vi "Check VI has Action Input.vi"(11 "Worker VI":refnum<vi>) -> (3 "Action Input?":bool)   [LabVIEW 2020, in "FlexBlock.xnode"]
uses:
  FlexBlock.xnode
  FlexBlocks/Worker Action.ctl
  FlexBlocks/FlexBlocks.lvlib
  <vilib>/Utility/Data Type/NI_Data Type.lvlib
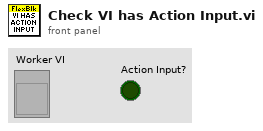
[diagram p1: front panel]
types:
  T1 = typedef "FlexBlocks.lvlib/Worker Action.ctl" = enum16{"Start", "Work", "Stop"}
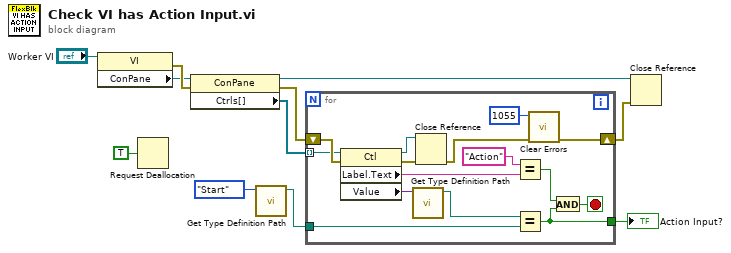
[diagram p0: block diagram]
diagram:
  n1 = property class="VI"(reference="Worker VI") -> (error out=w11:errorcluster, "ConPane"=w9:refnum<vi>)  [unwired: 1 in, 1 out]
  n2 = Request Deallocation(TRUE ("flag")) -> ()
  n3 = property class="ConPane"(reference=w9, error in=w11) -> (reference out=w4:refnum<vi>, error out=w7:errorcluster, "Ctrls[]"=w8:refnum<vi>[])
  n4 = call <vilib>:"Get Type Definition Path.vi"("variant"=Worker_Action."Start" ("Action")) -> ("type definition path"=w2:path)  [unwired: 9 in, 1 out]
  n5 = for {
    tunnel: w2 -> [w24]
    tunnel: w8 -> [w25] mode=indexing
    shift-right: [w13] -> w5
    shift-left: w7 -> [w26]
    tunnel: [w19] -> w6
    stop <- w17 stop-if-true
    n6 = property class="Ctl"(reference=w25, error in=w26) -> (reference out=w22:refnum<vi>, error out=w23:errorcluster, "Label.Text"=w21:string, "Value"=w16:variant)
    n7 = call <vilib>:"Get Type Definition Path.vi"("variant"=w16) -> ("type definition path"=w15:path)  [unwired: 9 in, 1 out]
    n8 = Close Reference(reference=w22, error in (no error)=w23) -> (error out=w14:errorcluster)
    n9 = Equal?(x="Action", y=w21) -> (x = y?=w18:bool)
    n10 = Equal?(x=w15, y=w24) -> (x = y?=w19:bool)
    n11 = call <vilib>:"Clear Errors.vi"("error in (no error)"=w14, "specific error code to clear (0: all)"=1055) -> ("error out"=w13:errorcluster)  [unwired: 4 in, 1 out]
    n12 = And(x=w18, y=w19) -> (x .and. y?=w17:bool)
  }
  "Action Input?" <- w6
  n13 = Close Reference(reference=w4, error in (no error)=w5) -> ()  [unwired: 1 out]
